vi "Multiple Connections - Client 1.vi"() -> ()   [LabVIEW 2011]
doc: "Establishes a connection to the specified host and port and reads the data and time data sent by the Server. The VI first reads 4 bytes defining the length of the date & time string and then reads the data. After you click the stop button, this VI sends a single character to tell the Date Server VI to terminate the connection.\n\n<B>Note:</B> Requires the use of theMultiple Connections - Server.vi."
panel:
  in  "string":string="00001:00002"
  in  "OK Button":bool
  in  "stop":bool
  in  "Machine":string="localhost"
  in  "Port":u16=6341
  # "Instructions:\n1. Open the Multiple Connections - Server.vi.\n2. Run the Multiple Connections - Server.vi first.\n3. Run the Client VIs second.\n4. Stop this VI and restart it to notice the # of Connections on the Server VI change.\n5. Stop the Server VI.  This VI will stop when it times out."
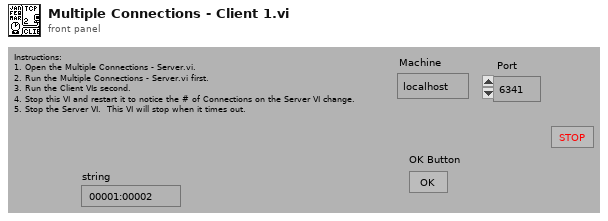
[diagram p1: front panel]
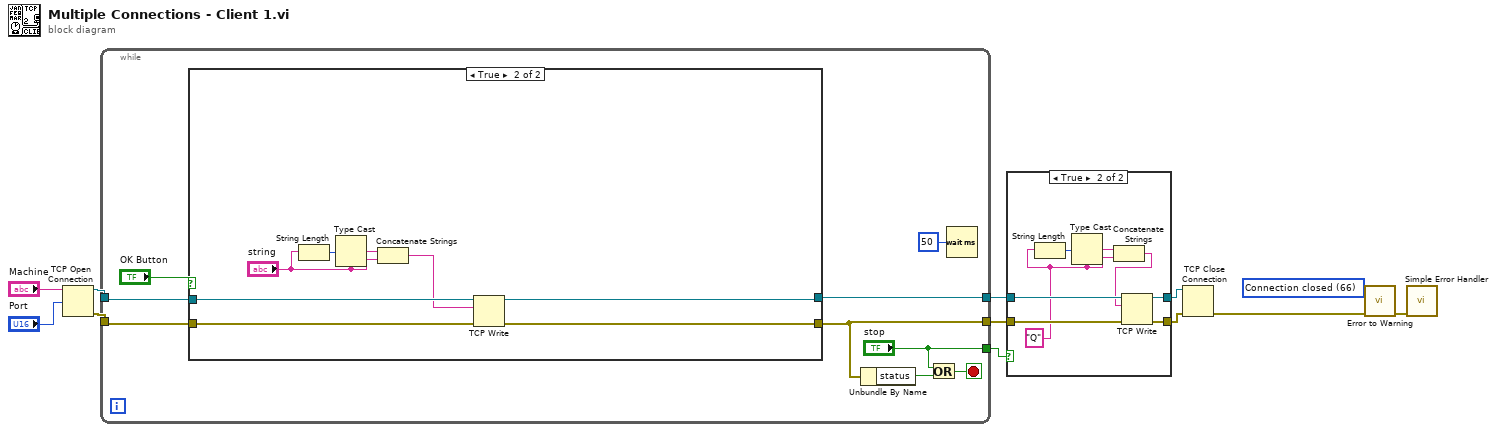
[diagram p0: block diagram]
diagram:
  w1 = 66 items=["No Error", "Argument Error", "Memory Full", "Out of Zone", "End of File", "File Already Open", "Generic File IO Error", "File Not Found", "File Permission Error", "Disk Full", "Duplicate Path", "Too Many Files Open", "Not Enabled", "Resource File Not Found", "Cannot Add Resource", "Resource Not Found", "Image Not Found", "Image Memory Error", "Pen Does Not Exist", "Config Bad Type", "Config Token Not Found", "Config Parse Error", "Config Memory Error", "Bad External Code Format", "Bad External Code Offset", "External Code Not Present", "Null Window", "Destroy Window Mixup", "Null Menu", "Print Aborted", "Bad Print Record", "Print Driver Error", "Windows Error During Print", "Memory Error During Print", "Print Dialog Error", "Generic Print Error", "Invalid Device Refnum", "Device Not Found", "Device Parameter Error", "Device Unit Error", "Can't Open Device", "Device Call Aborted", "Generic Error", "Cancelled By User", "Object ID Too Low", "Object ID Too High", "Object Not In Heap", "Unknown Heap", "Bad DefProc ID", "DefProc Not In Table", "Message Out Of Range", "Null Method", "Unknown Message", "Manager Call Not Supported", "Bad address", "Connection In progress", "Connection timed out", "Connection is already in progress", "Network attribute not supported", "Network error", "Address in use", "System out of memory", "Connection aborted", "Connection refused", "Connection is not connected", "Connection is already connected", "Connection closed", "Initialize error (interapplication manager)", "Bad occurrence", "Wait on unbound occurrence handler", "Occurrence queue overflow", "Bad path", "Semaphore not signaled", "Unrecognized type (interapplication manager)"] ("1st Error to Convert")
  n1 = TCP Open Connection(address="Machine", remote port or service name="Port") -> (connection ID=w10:refnum<k5>, error out=w9:errorcluster)  [unwired: 1 in, 2 out]
  n2 = while {
    tunnel: ["stop"] -> w4
    tunnel: [w14] -> w8
    tunnel: [w15] -> w6
    tunnel: w9 -> [w16]
    tunnel: w10 -> [w17]
    stop <- w21 stop-if-true
    n3 = case shown="True" "OK Button" {
      tunnel: w17 -> [w23 w31]
      tunnel: w16 -> [w22 w30]
      tunnel: [w22 w24] -> w15
      tunnel: [w23 w25] -> w14
      frame False {
      }
      frame True {
        n4 = String Length(string="string") -> (length=w29:i32)
        n5 = Type Cast(type="string", x=w29) -> (*(type *) &x=w28:string)
        n6 = Concatenate Strings(w28, "string") -> (w27:string)
        n7 = TCP Write(connection ID=w31, data in=w27, error in (no error)=w30) -> (connection ID out=w25:refnum<k5>, error out=w24:errorcluster)  [unwired: 1 in, 1 out]
      }
    }
    n8 = Unbundle By Name(w15) -> ("status"=w20:bool)
    n9 = Or(x="stop", y=w20) -> (x .or. y?=w21:bool)
    n10 = Wait (ms)(milliseconds to wait=u32 50) -> ()  [unwired: 1 out]
  }
  n11 = case shown="True" w4 {
    tunnel: w8 -> [w33 w41]
    tunnel: [w33 w39] -> w7
    tunnel: w6 -> [w32 w40]
    tunnel: [w32 w38] -> w5
    frame False {
    }
    frame True {
      w35 = "Q"
      n12 = String Length(string=w35) -> (length=w37:i32)
      n13 = Type Cast(type=w35, x=w37) -> (*(type *) &x=w36:string)
      n14 = Concatenate Strings(w36, w35) -> (w34:string)
      n15 = TCP Write(connection ID=w41, data in=w34, error in (no error)=w40) -> (connection ID out=w39:refnum<k5>, error out=w38:errorcluster)  [unwired: 2 out]
    }
  }
  n16 = TCP Close Connection(connection ID=w7, error in (no error)=w5) -> (error out=w3:errorcluster)  [unwired: 2 out]
  n17 = call <vilib>:"Error to Warning.vi"("1st Error to Convert"=w1, "error in"=w3) -> ("warning out"=w2:errorcluster)  [unwired: 3 in, 10 out]
  n18 = call <vilib>:"Simple Error Handler.vi"("error in (no error)"=w2) -> ()  [unwired: 1 in, 8 out]
